vi "forward_Akhilesh.vi"() -> ()   [LabVIEW 2019]
uses:
  Control 7.ctl
panel:
  in  "Boolean":bool
  in  "Boolean 2":bool
  in  "stop":bool
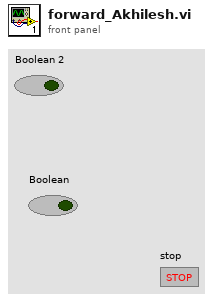
[diagram p1: front panel]
types:
  T1 = typedef "Control 7.ctl" = enum16{"Forward", "Turn"}
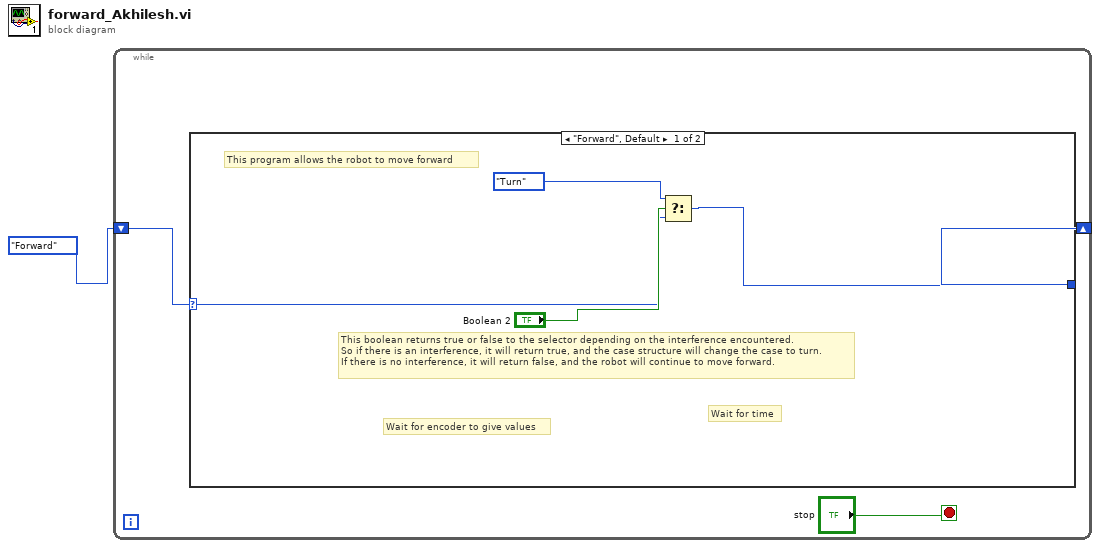
[diagram p0: block diagram]
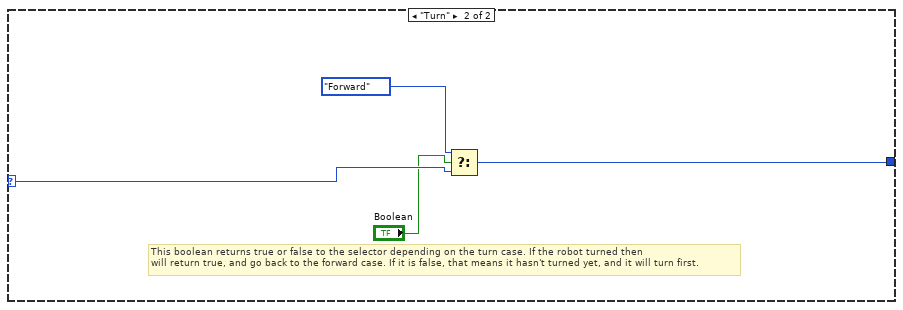
[diagram p2: hidden frame]
diagram:
  n1 = while {
    shift-right: [w3] -> _
    shift-left: Control_7."Forward" -> [w2]
    stop <- "stop" stop-if-true
    n2 = case shown="\"Forward\", Default" w2 {
      selector: w2 -> [w6 w12]
      tunnel: [w8 w11] -> w3
      frame "Forward", Default {
        # "Wait for time"
        # "Wait for encoder to give values"
        # "This boolean returns true or false to the selector depending on the interference encountered.\nSo if there is an interference, it will return true, and the case structure will change the case to turn.\nIf there is no interference, it will return false, and the robot will continue to move forward."
        # "This program allows the robot to move forward"
        n3 = Select(t=Control_7."Turn", s="Boolean 2", f=w6) -> (s? t:f=w8:T1)
      }
      frame "Turn" {
        # "This boolean returns true or false to the selector depending on the turn case. If the robot turned then \nwill return true, and go back to the forward case. If it is false, that means it hasn't turned yet, and it will turn first."
        n4 = Select(t=Control_7."Forward", s="Boolean", f=w12) -> (s? t:f=w11:T1)
      }
    }
  }
